vi "Read Destination IP.vi"(8 "error in (no error)":errorcluster, 11 "TCP Listener in":refnum<class "TCP Listener.lvclass">) -> (0 "error out":errorcluster, 2 "Destination IP":string, 3 "TCP Listener out":refnum<class "TCP Listener.lvclass">)   [LabVIEW 2026, in "TALOS.lvlib" / "TCP Listener.lvlib" / "TCP Listener.lvclass"]
uses:
  TCP Listener.lvclass
  TCP Listener.lvclass/TCP Listener.ctl
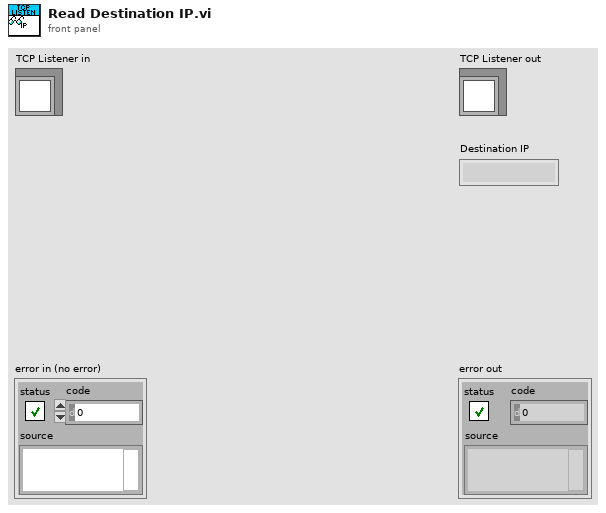
[diagram p1: front panel]
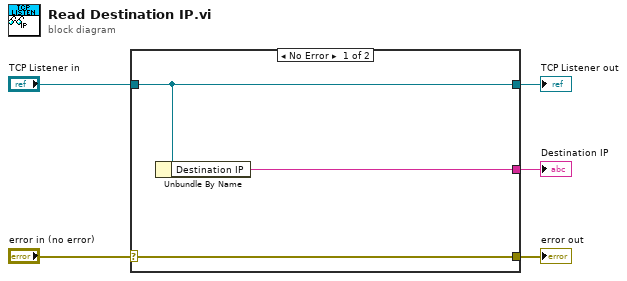
[diagram p0: block diagram]
diagram:
  n1 = case shown="No Error" "error in (no error)" {
    selector: "error in (no error)" -> [w8 w9]
    tunnel: [w8 w9] -> w4
    tunnel: [w7 w10] -> w2
    tunnel: "TCP Listener in" -> [w7 w10]
    tunnel: [w6 _] -> w1
    frame No Error {
      n2 = Unbundle By Name(w7) -> ("Destination IP"=w6:string)
    }
    frame Error {
    }
  }
  "error out" <- w4
  "TCP Listener out" <- w2
  "Destination IP" <- w1
